vi "SUB_SyncroCondition.vi"(4 "DelayIn":dbl, 5 "Condition":T1, 6 "TaskRead In":refnum<k21>, 7 "TaskWrite In":refnum<k21>) -> (0 "DelayOut":dbl, 1 "TaskWrite Out":refnum<k21>, 2 "TaskRead Out":refnum<k21>, 3 "error out":errorcluster)   [LabVIEW 2015]
uses:
  <vilib>/DAQmx/configure/trigger.llb/DAQmx Start Trigger (Analog Edge).vi
  <vilib>/DAQmx/configure/trigger.llb/DAQmx Start Trigger (Digital Edge).vi
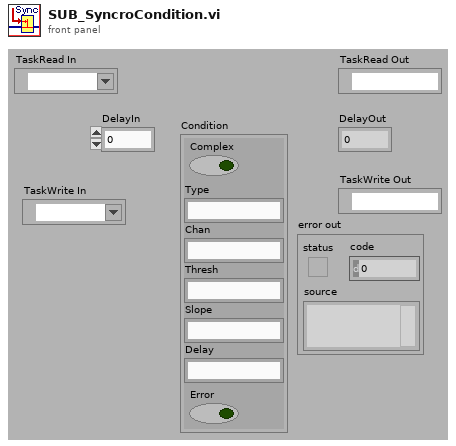
[diagram p1: front panel]
types:
  T1 = cluster{"Complex":bool, "Type":string, "Chan":string, "Thresh":string, "Slope":string, "Delay":string, "Error":bool}
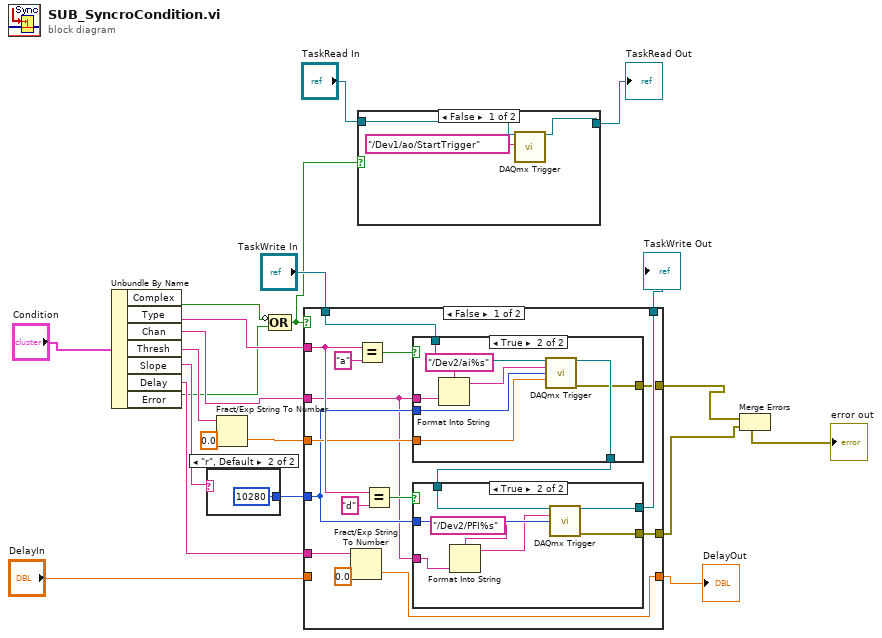
[diagram p0: block diagram]
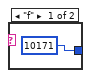
[diagram p3: hidden frame]
diagram:
  n1 = Unbundle By Name("Condition") -> ("Complex"=w11:bool, "Type"=w12:string, "Chan"=w21:string, "Thresh"=w14:string, "Slope"=w16:string, "Delay"=w20:string, "Error"=w10:bool)
  n2 = case shown="\"r\", Default" w16 {
    tunnel: [10171 10280] -> w17
    frame "f" {
    }
    frame "r", Default {
    }
  }
  n3 = Fract/Exp String To Number(string=w14, default (0 dbl)=0.0) -> (number=w15:dbl)  [unwired: 3 out]
  n4 = Compound Arithmetic op=OR(invert w11, w10) -> (w1:bool)
  n5 = case shown="False" w1 {
    tunnel: [w29 w57] -> w7
    tunnel: w12 -> [w35 _]
    tunnel: w15 -> [w33 _]
    tunnel: w21 -> [w27 _]
    tunnel: w17 -> [w28 _]
    tunnel: "DelayIn" -> [_ w58]
    tunnel: [w30 w58] -> w19
    tunnel: w20 -> [w31 _]
    tunnel: "TaskWrite In" -> [w26 w57]
    tunnel: [w25 _] -> w2
    tunnel: [w24 _] -> w3
    frame False {
      n6 = Fract/Exp String To Number(string=w31, default (0 dbl)=0.0) -> (number=w30:dbl)  [unwired: 3 out]
      n7 = Equal?(x=w35, y="a") -> (x = y?=w38:bool)
      n8 = Equal?(x=w35, y="d") -> (x = y?=w36:bool)
      n9 = case shown="True" w38 {
        tunnel: w26 -> [w48 w56]
        tunnel: [w48 w55] -> w34
        tunnel: w33 -> [_ w54]
        tunnel: w27 -> [_ w51]
        tunnel: w28 -> [_ w53]
        tunnel: [_ w49] -> w24
        frame False {
        }
        frame True {
          n10 = Format Into String(format string="/Dev2/ai%s", w51) -> (resulting string=w50:string)  [unwired: 2 in, 1 out]
          n11 = call-poly <vilib>:"DAQmx Trigger.vi"("task/channels in"=w56, "source"=w50, "slope"=w53, "level"=w54) -> ("task out"=w55:refnum<k21>, "error out"=w49:errorcluster)  [unwired: 1 in, 9 out]
        }
      }
      n12 = case shown="True" w36 {
        tunnel: w34 -> [w40 w47]
        tunnel: [w40 w46] -> w29
        tunnel: w28 -> [_ w45]
        tunnel: w27 -> [_ w44]
        tunnel: [_ w41] -> w25
        frame False {
        }
        frame True {
          n13 = Format Into String(format string="/Dev2/PFI%s", w44) -> (resulting string=w43:string)  [unwired: 2 in, 1 out]
          n14 = call-poly <vilib>:"DAQmx Trigger.vi"("task/channels in"=w47, "source"=w43, "edge"=w45) -> ("task out"=w46:refnum<k21>, "error out"=w41:errorcluster)  [unwired: 1 in, 10 out]
        }
      }
    }
    frame True {
      # "If error in trigger definition or simple trigger is defined"
    }
  }
  "DelayOut" <- w19
  "TaskWrite Out" <- w7
  n15 = case shown="False" w1 {
    tunnel: [w61 w62] -> w5
    tunnel: "TaskRead In" -> [w60 w62]
    frame False {
      n16 = call-poly <vilib>:"DAQmx Trigger.vi"("task/channels in"=w60, "source"=tag "/Dev1/ao/StartTrigger") -> ("task out"=w61:refnum<k21>)  [unwired: 2 in, 11 out]
    }
    frame True {
    }
  }
  "TaskRead Out" <- w5
  n17 = Merge Errors(w3, w2) -> (→"error out":errorcluster)
